vi "GPS.vi"() -> ()   [LabVIEW 2015]
uses:
  <vilib>/Instr/_visa.llb/VISA Configure Serial Port (Instr).vi
panel:
  out "Number of satellites in use":dbl
  out "Longitude [deg]":string
  out "Latitude [deg]":string
  out "Time":string
  in  "Time zone":i32
  out "Mode":string
  out "Date [ddmmyy]":string
  out "Course over ground [degrees]":string
  out "Speed over ground (knots)":string
  out "E/W":string
  out "Longitude":string
  out "N/S":string
  out "Latitude":string
  out "Status":string
  out "UTC Time":string
  out "NMEA Sentances":string
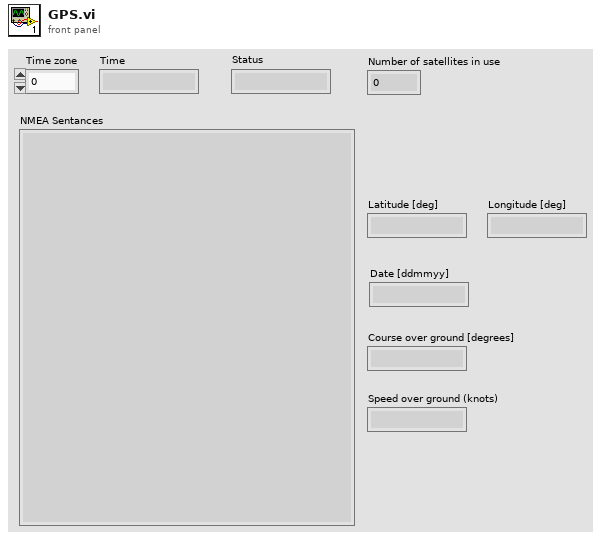
[diagram p1: front panel]
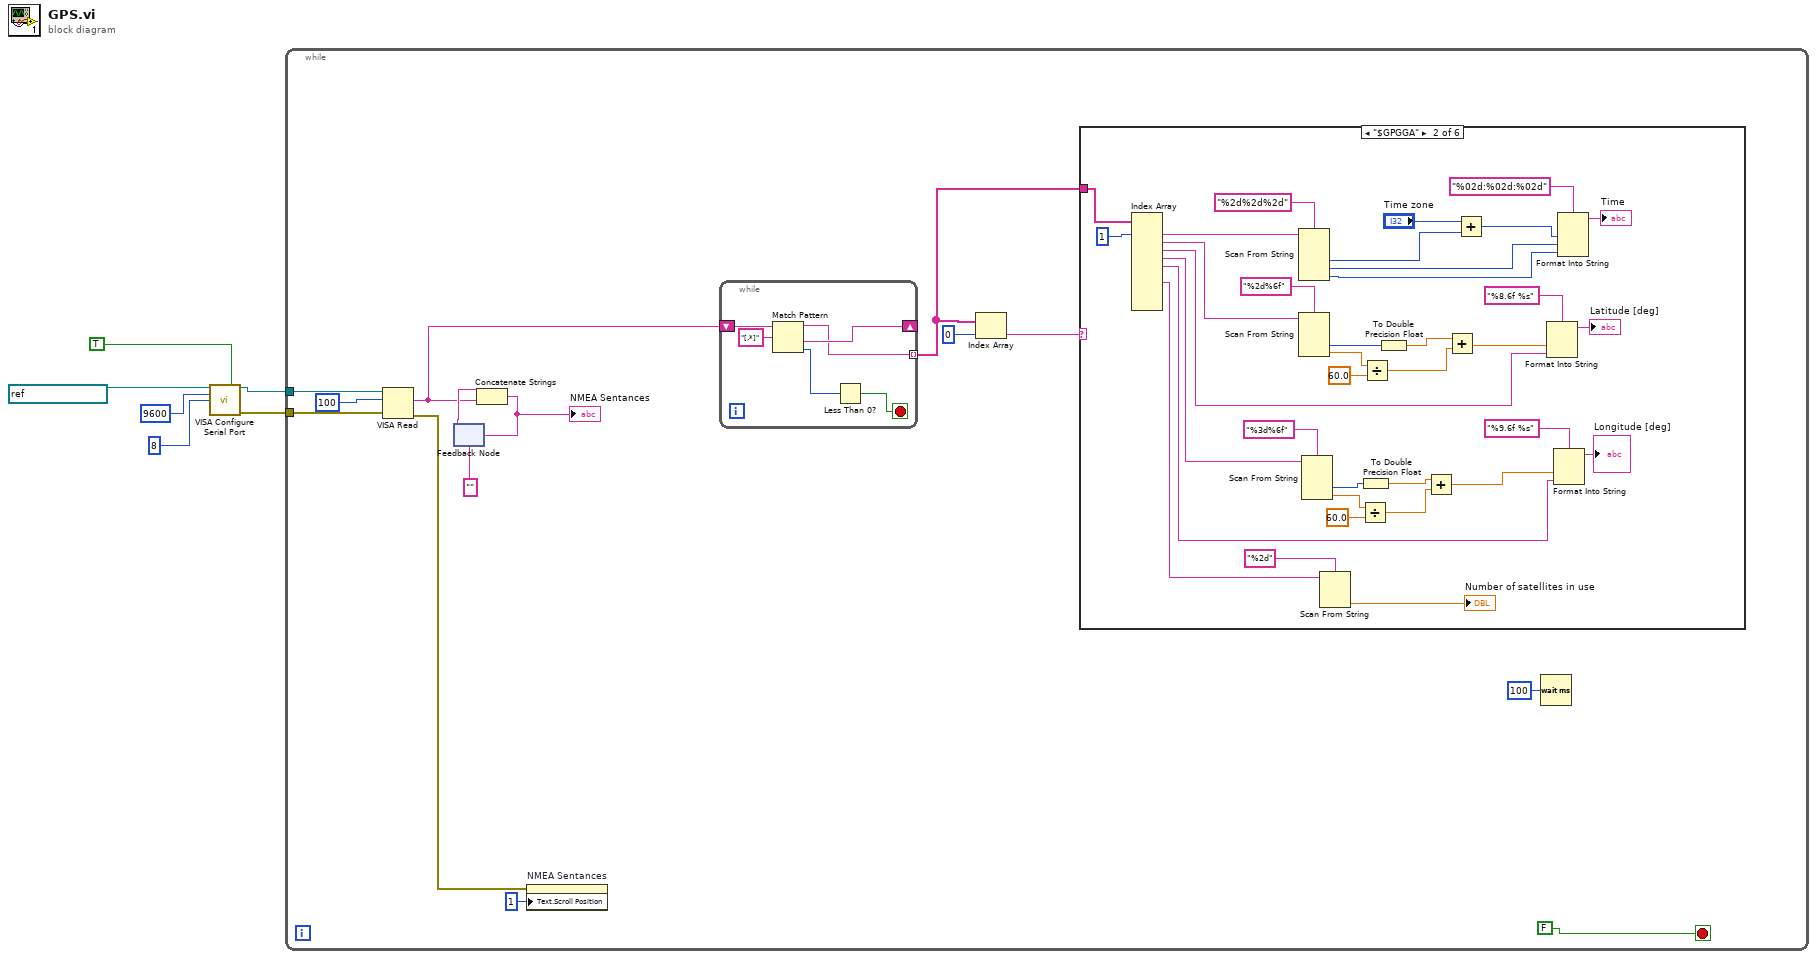
[diagram p0: block diagram]
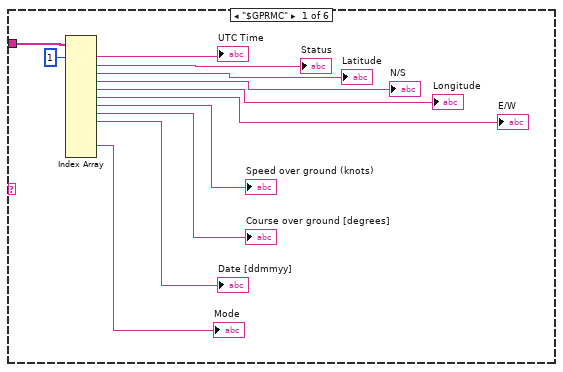
[diagram p2: hidden frame]
diagram:
  n1 = call-poly "VISA Configure Serial Port"("VISA resource name"=refnum<visa-resource-name> "ASRL1::INSTR", "Enable Termination\nChar (T)"=TRUE ("Enable Termination\nChar (T)"), "baud rate (9600)"=u32 9600, "data bits (8)"=u16 8) -> ("VISA resource name out"=w2:refnum<visa-resource-name>, "error out"=w1:errorcluster)  [unwired: 10 in]
  n2 = while {
    tunnel: w2 -> [w20]
    tunnel: w1 -> [w19]
    stop <- FALSE stop-if-true
    n3 = VISA Read(VISA resource name=w20, byte count=u32 100, error in (no error)=w19) -> (read buffer=w12:string, error out=w14:errorcluster)  [unwired: 2 out]
    n4 = feedback #1("") -> (w16:string)
    n5 = Concatenate Strings "Concatenate Strings"(w16, w12) -> (w17:string)
    "NMEA Sentances" <- w17
    n6 = feedback-in #1(w17) -> ()
    n7 = property on="NMEA Sentances" class="Str"(error in=w14, "Text.Scroll Position"=u32 1) -> ()  [unwired: 1 in, 2 out]
    n8 = while {
      shift-right: [w70] -> _
      shift-left: w12 -> [w74]
      tunnel: [w69] -> w9 mode=indexing
      stop <- w72 stop-if-true
      n9 = Match Pattern(string=w74, regular expression="[,*]") -> (before substring=w69:string, after substring=w70:string, offset past match=w71:i32)  [unwired: 1 in, 1 out]
      n10 = Less Than 0?(x=w71) -> (x < 0?=w72:bool)
    }
    n11 = Index Array(array=w9, index=0) -> (element=w10:string)
    n12 = case shown="\"$GPGGA\"" w10 {
      tunnel: w9 -> [w31 w68 _ _ _ _]
      frame "$GPRMC" {
        n13 = Index Array(array=w31, index #1=1 ("index")) -> (element #1=→"UTC Time":string, element #2=→"Status":string, element #3=→"Latitude":string, element #4=→"N/S":string, element #5=→"Longitude":string, element #6=→"E/W":string, element #7=→"Speed over ground (knots)":string, element #8=→"Course over ground [degrees]":string, element #9=→"Date [ddmmyy]":string, element #12=→"Mode":string)  [unwired: 12 in, 3 out]
      }
      frame "$GPGGA" {
        n14 = Index Array(array=w68, index #1=1 ("index")) -> (element #1=w66:string, element #2=w56:string, element #3=w48:string, element #4=w45:string, element #5=w39:string, element #7=w35:string)  [unwired: 9 in, 4 out]
        n15 = Scan From String(format string="%2d%2d%2d", input string=w66) -> (output 1=w64:i32, output 2=w61:i32, output 3=w58:i32)  [unwired: 5 in, 3 out]
        n16 = Scan From String(format string="%2d%6f", input string=w56) -> (output 1=w55:i32, output 2=w53:dbl)  [unwired: 4 in, 3 out]
        n17 = Scan From String(format string="%3d%6f", input string=w45) -> (output 1=w44:i32, output 2=w41:dbl)  [unwired: 4 in, 3 out]
        n18 = Scan From String(format string="%2d", input string=w35) -> (output 1=→"Number of satellites in use":dbl)  [unwired: 3 in, 3 out]
        n19 = Divide(x=w41, y=60.0) -> (x/y=w40:dbl)
        n20 = To Double Precision Float(number=w44) -> (double precision float=w43:dbl)
        n21 = Divide(x=w53, y=60.0) -> (x/y=w52:dbl)
        n22 = To Double Precision Float(number=w55) -> (double precision float=w51:dbl)
        n23 = Add(x=w43, y=w40) -> (x+y=w38:dbl)
        n24 = Add(x=w51, y=w52) -> (x+y=w49:dbl)
        n25 = Add(x="Time zone", y=w64) -> (x+y=w62:i32)
        n26 = Format Into String(format string="%8.6f %s", w49, w48) -> (resulting string=→"Latitude [deg]":string)  [unwired: 2 in, 1 out]
        n27 = Format Into String(format string="%9.6f %s", w38, w39) -> (resulting string=→"Longitude [deg]":string)  [unwired: 2 in, 1 out]
        n28 = Format Into String(format string="%02d:%02d:%02d", w62, w61, w58) -> (resulting string=→"Time":string)  [unwired: 2 in, 1 out]
      }
      frame "GPGSA" {
      }
      frame "$GPGSV" {
      }
      frame "$GPVTG" {
      }
      frame Default {
      }
    }
    n29 = Wait (ms)(milliseconds to wait=u32 100) -> ()  [unwired: 1 out]
  }
